vi "Select stimulus.vi"(10 "Output freq (Hz)":dbl=50.0) -> (0 "cancelled":bool, 1 "stimphases":T1, 2 "output waveform":waveform(dbl), 3 "Stimulus":T2={"type"=enum."Zero", "sinfreq start"=0.0, "sinfreq end"=0.0, "sinamp start"=0.0, "sinamp end"=0.0, "noise freq lo"=0.0, "noise freq hi"=0.0, "noiseamp start"=0.0, "noiseamp end"=0.0, "stimdur"=100.0, "before dur"=20.0, "after dur"=30.0, "pulse data"={"time"=[], "phase/vel"=[], "dir/shift"=[], "amplitude"=[], "duration"=[]}} {"noise freq hi" min=0.0 step=0.5; "noise freq lo" min=0.0 step=0.5; "noiseamp end" min=0.0 step=0.5; "noiseamp start" min=0.0 step=0.5})   [LabVIEW 2013]
uses:
  Stimulus.ctl
  Stimulus type.ctl
  Pulse data.ctl
  Stim phases.ctl
panel:
  in  "offset":dbl[unit] caption="Offset"
  out "Waveform Graph":waveform(dbl)[](graph)=[{"t0"=timestamp(0 s since 1904-01-01), "dt"=inf, "Y"=[]}, {"t0"=timestamp(0 s since 1904-01-01), "dt"=inf, "Y"=[]}, {"t0"=timestamp(0 s since 1904-01-01), "dt"=inf, "Y"=[]}]
  in  "Cancel":bool
  in  "OK":bool
  in  "Stimulus type":T5(tab)=enum."Frequency sweep"
  in  "stimdurzero":dbl=100.0 caption="Stimulus"
  in  "stimdursin":dbl=100.0 caption="Stimulus"
  in  "beforesin":dbl[unit]=20.0 caption="Before"
  in  "aftersin":dbl[unit]=30.0 caption="After"
  in  "noisehifreq":dbl[unit]=10.0 caption="High cutoff" format="%#_10g"
  in  "noiseamp":dbl[unit] caption="Amplitude"
  in  "noiselofreq":dbl[unit] caption="Low cutoff"
  in  "sinamp":dbl[unit]=0.3490658503988659 caption="Amplitude"
  in  "sinfreq":dbl[unit]=1.0 caption="Frequency" format="%#_10g"
  in  "stimdurampsweep":dbl=100.0 caption="Stimulus"
  in  "Hi freq cutoff":dbl[unit]=10.0 min=0.0 step=0.5
  in  "Lo freq cutoff":dbl[unit] min=0.0 step=0.5
  in  "Start noise":dbl[unit] caption="Start" min=0.0 step=0.008726646259971648
  in  "Frequency":dbl[unit]=1.0 min=0.0 step=0.05
  in  "Start amp":dbl[unit]=0.5235987755982988 caption="Start" min=0.0 step=0.017453292519943295
  in  "End amplitude":dbl[unit]=0.5235987755982988 caption="End" min=0.0 step=0.017453292519943295
  in  "End noise":dbl[unit] caption="End" min=0.0 step=0.008726646259971648
  in  "beforeampsweep":dbl[unit]=20.0 caption="Before"
  in  "afterampsweep":dbl[unit]=30.0 caption="After"
  in  "stimdurfreqsweep":dbl=100.0 caption="Stimulus"
  in  "beforefreqsweep":dbl[unit]=20.0 caption="Before"
  in  "afterfreqsweep":dbl[unit]=30.0 caption="After"
  in  "hi cutoff":dbl[unit]=10.0 caption="High cutoff"
  in  "noiseamp":dbl[unit] caption="Amplitude"
  in  "lo cutoff":dbl[unit] caption="Low cutoff"
  in  "endfreq":dbl[unit]=2.0 caption="End" min=0.0 step=0.05
  in  "startfreq":dbl[unit]=0.5 caption="Start" min=0.0 step=0.05
  in  "sinamp":dbl=30.0 caption="Amplitude" min=0.0 step=1.0
  in  "beforepulses":dbl[unit]=20.0 caption="Before"
  in  "afterpulses":dbl[unit]=30.0 caption="After"
  in  "precycles":dbl=1.0 caption="Initial cycles"
  out "totaltime":dbl caption="Total time"
  in  "cyclesperpulse":dbl=1.0 caption="Cycles per pulse"
  in  "pulsedur":dbl[unit]=0.02 caption="Duration"
  in  "pulseamp":dbl[unit]=0.3490658503988659 caption="Amplitude"
  in  "pulsedir":enum16{"Left", "Right", "Both"}(ring) caption="Direction"
  in  "randomphase":bool
  in  "phases":i32=1 caption="Number of phases"
  in  "pulsereps":i32=1 caption="Repetitions"
  in  "sinamp":dbl[unit]=0.3490658503988659 caption="Amplitude"
  in  "sinfreq":dbl[unit]=1.0 caption="Frequency"
  in  "rampdir":enum16{"Left", "Right", "Both"}(ring)=enum."Both" caption="Direction"
  in  "Hold time (s)":dbl[](array[numeric])=[0.0, 10.0]
  out "Total time":dbl[unit]
  in  "Randomize":bool=TRUE
  in  "Repetitions":i32=1 min=0 step=1
  in  "Final positions (deg)":dbl[](array[numeric])=[2.0, 5.0, 10.0]
  in  "Ramp velocities (deg/s)":dbl[](array[numeric])=[1.0, 10.0]
  in  "gap time (s)":dbl=5.0 min=0.0 step=0.5
  in  "beforeramps":dbl[unit]=20.0 caption="Before"
  in  "afterramps":dbl[unit]=30.0 caption="After"
  in  "beforeshifts":dbl[unit]=20.0 caption="Before"
  in  "aftershifts":dbl[unit]=30.0 caption="After"
  in  "endphases":i32=1 caption="Number of ending phases"
  in  "precycles":dbl=1.0 caption="Initial cycles"
  out "totaltime":dbl caption="Total time"
  in  "cyclespershift":dbl=1.0 caption="Cycles per stim"
  in  "shiftdur":dbl[unit]=0.02 caption="Duration"
  in  "randomize":bool
  in  "startphases":i32=1 caption="Number of starting phases"
  in  "shiftreps":i32=1 caption="Repetitions"
  in  "sinamp":dbl[unit]=0.3490658503988659 caption="Amplitude"
  in  "sinfreq":dbl[unit]=1.0 caption="Frequency"
  # "Just record baseline bursting with no stimulus"
  # "Duration:"
  # "s"
  # "Signal:"
  # "Noise:"
  # "Duration:"
  # "cycles"
  # "Signal:"
  # "Amplitude:"
  # "Noise:"
  # "Amplitude:"
  # "Duration:"
  # "cycles"
  # "Signal:"
  # "Frequency:"
  # "Noise:"
  # "Duration:"
  # "s"
  # "Signal:"
  # "Pulses:"
  # "Duration:"
  # "Signal:"
  # "Shifts:"
  # "Duration:"
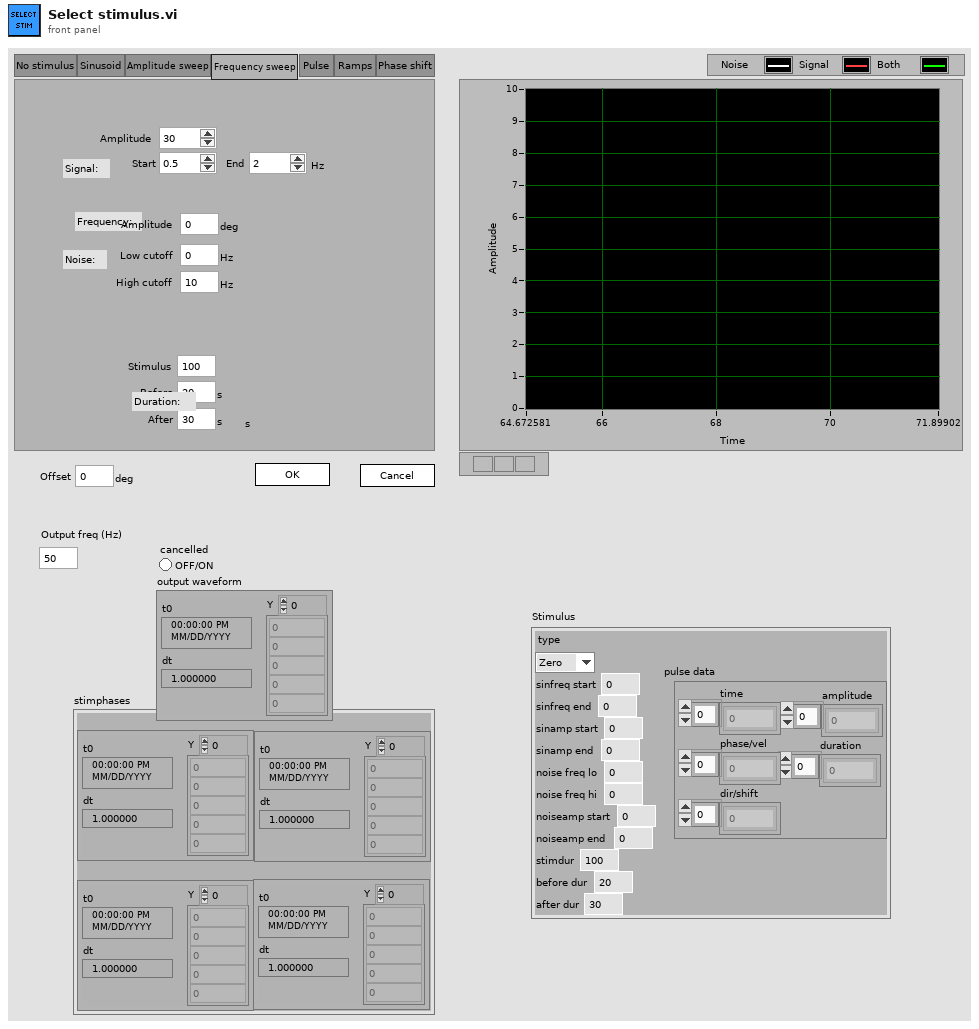
[diagram p1: front panel]
types:
  T1 = typedef "Stim phases.ctl" = cluster{"sinephase":waveform(dbl), "sinecycles":waveform(dbl), "stimphase":waveform(dbl), "stimcycles":waveform(dbl)}
  T2 = typedef "Stimulus.ctl" = cluster{"type":T3, "sinfreq start":dbl, "sinfreq end":dbl, "sinamp start":dbl, "sinamp end":dbl, "noise freq lo":dbl, "noise freq hi":dbl, "noiseamp start":dbl, "noiseamp end":dbl, "stimdur":dbl, "before dur":dbl, "after dur":dbl, "pulse data":T4}
  T3 = typedef "Stimulus type.ctl" = enum16{"Sine", "Zero", "Frequency sweep", "Two frequency", "Amplitude sweep", "Pulses", "Shifts", "Ramps"}
  T4 = typedef "Pulse data.ctl" = cluster{"time":dbl[], "phase/vel":dbl[], "dir/shift":dbl[], "amplitude":dbl[], "duration":dbl[]}
  T5 = enum32{"No stimulus", "Sinusoid", "Amplitude sweep", "Frequency sweep", "Pulse", "Ramps", "Phase shift"}
  T6 = typedef "Phases.ctl" = cluster{"sinephase":dbl[], "sinecycle":dbl[], "stimphase":dbl[], "stimcycle":dbl[]}
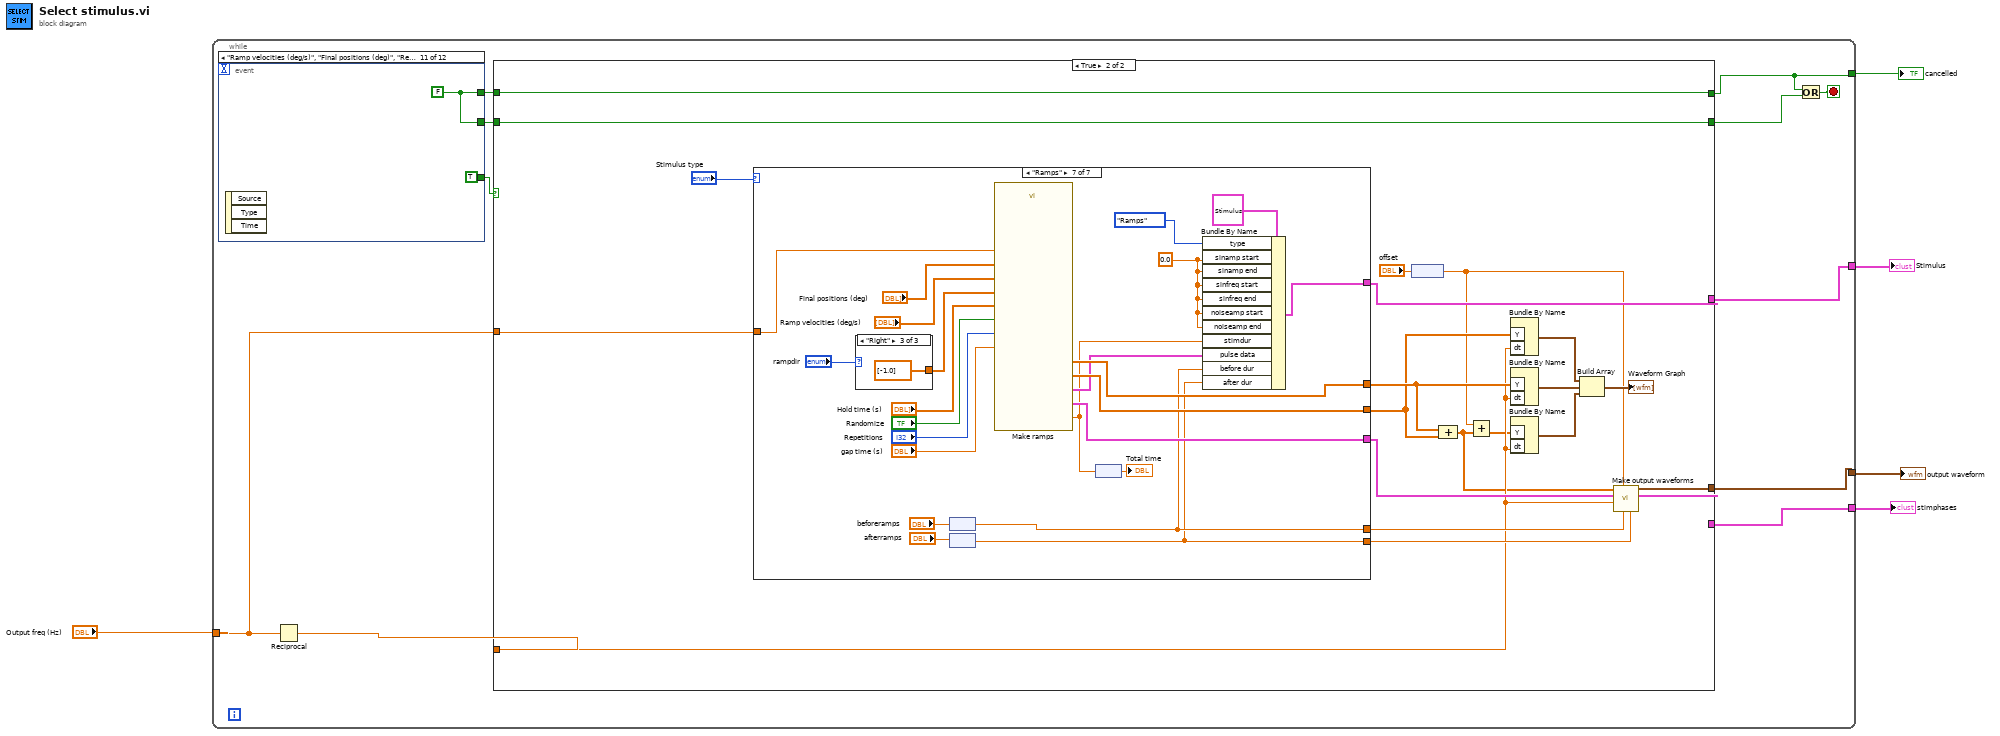
[diagram p0: block diagram]
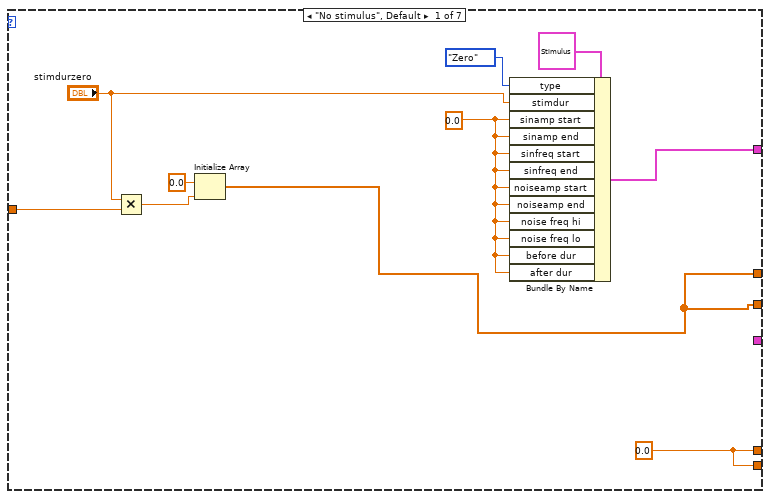
[diagram p3: hidden frame]
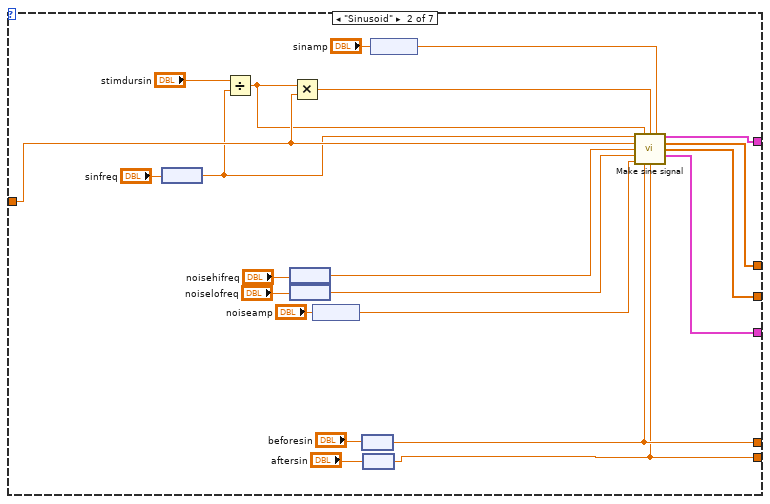
[diagram p4: hidden frame]
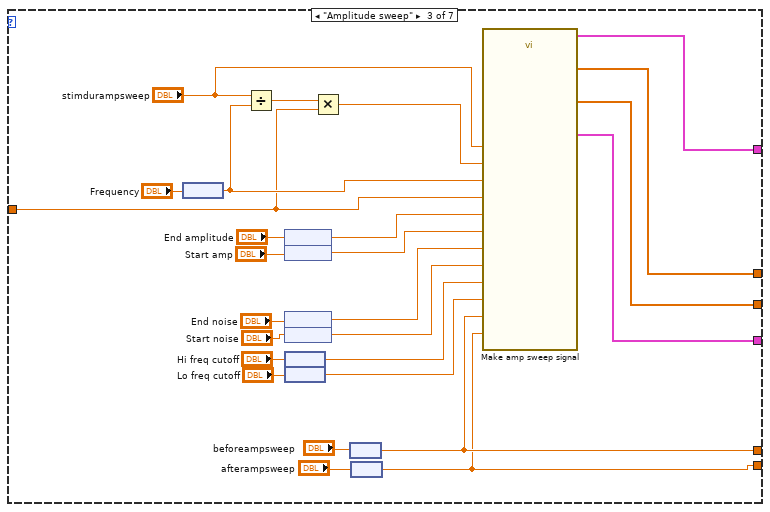
[diagram p5: hidden frame]
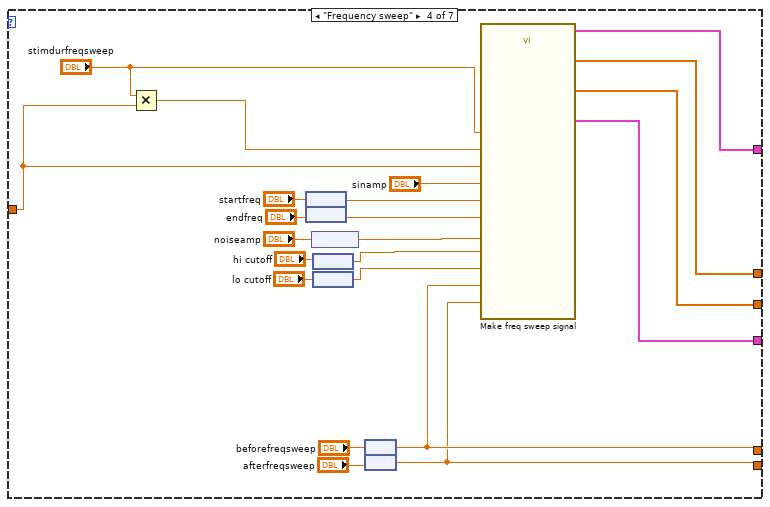
[diagram p6: hidden frame]
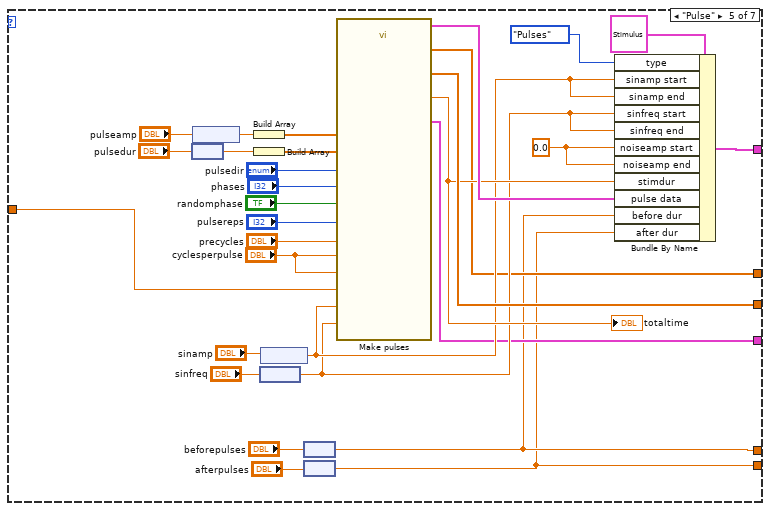
[diagram p7: hidden frame]
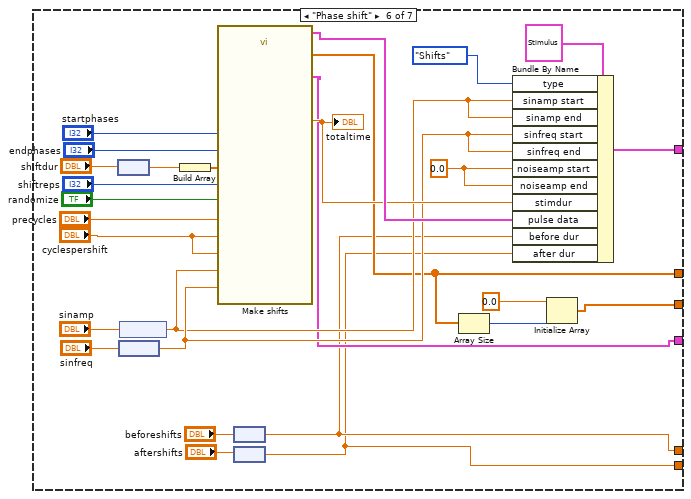
[diagram p8: hidden frame]
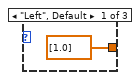
[diagram p9: hidden frame]
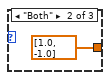
[diagram p10: hidden frame]
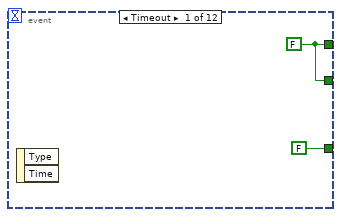
[diagram p11: hidden frame]
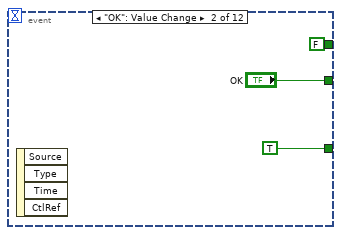
[diagram p12: hidden frame]
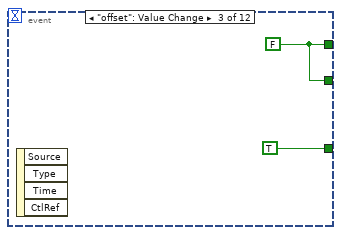
[diagram p13: hidden frame]
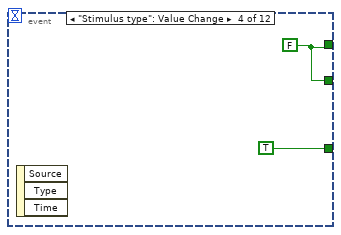
[diagram p14: hidden frame]
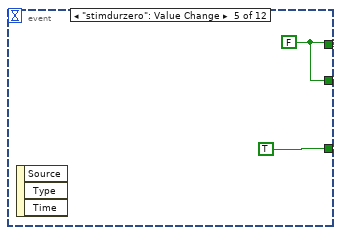
[diagram p15: hidden frame]
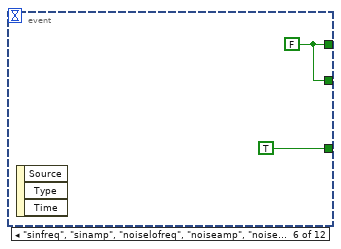
[diagram p16: hidden frame]
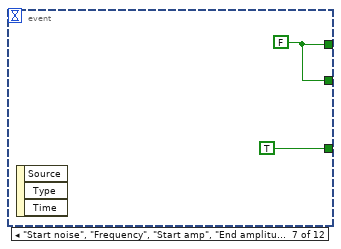
[diagram p17: hidden frame]
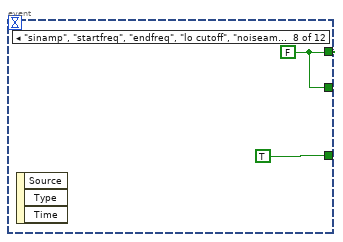
[diagram p18: hidden frame]
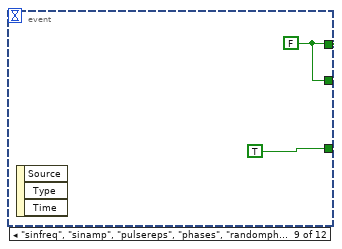
[diagram p19: hidden frame]
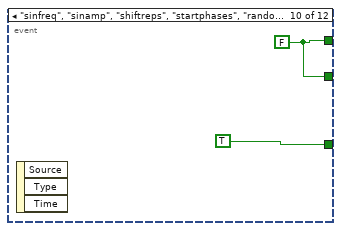
[diagram p20: hidden frame]
diagram:
  n1 = while {
    tunnel: "Output freq (Hz)" -> [w16]
    tunnel: [w7] -> w4
    tunnel: [w14] -> w3
    tunnel: [w13] -> w2
    tunnel: [w12] -> w1
    stop <- w11 stop-if-true
    n2 = event shown="[10] \"Ramp velocities (deg/s)\", \"Final positions (deg)\", \"Repetitions\", \"Randomize\", \"Hold time (s)\", \"rampdir\", \"gap time (s)\", \"beforeramps\", \"afterramps\": Value Change" {
      selector: _ -> [_ _ _ _ _ _ _ _ _ _ _ _]
      dyn-events: _ -> [_ _ _ _ _ _ _ _ _ _ _ _]
      timeout: _ -> [_ _ _ _ _ _ _ _ _ _ _ _]
      tunnel: [FALSE TRUE TRUE TRUE TRUE TRUE TRUE TRUE TRUE TRUE TRUE FALSE] -> w6
      tunnel: [w204 "OK" w209 w211 w213 w215 w217 w219 w221 w223 w226 FALSE] -> w10
      tunnel: [w204 FALSE ("Cancel") w209 w211 w213 w215 w217 w219 w221 w223 w226 "Cancel"] -> w8
      event Timeout {
        w204 = FALSE
        n3 = event-data() -> ()  [unwired: 1 in, 2 out]
      }
      event "OK": Value Change {
        n4 = event-data() -> ()  [unwired: 1 in, 4 out]
      }
      event "offset": Value Change {
        w209 = FALSE ("Cancel")
        n5 = event-data() -> ()  [unwired: 1 in, 4 out]
      }
      event "Stimulus type": Value Change {
        w211 = FALSE
        n6 = event-data() -> ()  [unwired: 1 in, 3 out]
      }
      event "stimdurzero": Value Change {
        w213 = FALSE
        n7 = event-data() -> ()  [unwired: 1 in, 3 out]
      }
      event "sinfreq", "sinamp", "noiselofreq", "noiseamp", "noisehifreq", "Hi freq cutoff", "Lo freq cutoff": Value Change {
        w215 = FALSE
        n8 = event-data() -> ()  [unwired: 1 in, 3 out]
      }
      event "Start noise", "Frequency", "Start amp", "End amplitude", "End noise": Value Change {
        w217 = FALSE
        n9 = event-data() -> ()  [unwired: 1 in, 3 out]
      }
      event "sinamp", "startfreq", "endfreq", "lo cutoff", "noiseamp", "hi cutoff": Value Change {
        w219 = FALSE
        n10 = event-data() -> ()  [unwired: 1 in, 3 out]
      }
      event "sinfreq", "sinamp", "pulsereps", "phases", "randomphase", "pulsedir", "pulseamp", "pulsedur", "cyclesperpulse", "precycles": Value Change {
        w221 = FALSE
        n11 = event-data() -> ()  [unwired: 1 in, 3 out]
      }
      event "sinfreq", "sinamp", "shiftreps", "startphases", "randomize", "shiftdur", "cyclespershift", "precycles", "endphases": Value Change {
        w223 = FALSE
        n12 = event-data() -> ()  [unwired: 1 in, 3 out]
      }
      event "Ramp velocities (deg/s)", "Final positions (deg)", "Repetitions", "Randomize", "Hold time (s)", "rampdir", "gap time (s)", "beforeramps", "afterramps": Value Change {
        w226 = FALSE ("Cancel")
        n13 = event-data() -> ()  [unwired: 1 in, 3 out]
      }
      event "Cancel": Value Change {
        n14 = event-data() -> ()  [unwired: 1 in, 5 out]
      }
    }
    n15 = Reciprocal(x=w16) -> (1/x=w15:dbl)
    n16 = case shown="True" w6 {
      tunnel: w16 -> [_ w32]
      tunnel: w15 -> [_ w28]
      tunnel: [_ w27] -> w14
      tunnel: [_ w26] -> w13
      tunnel: [_ w25] -> w12
      tunnel: w10 -> [w17 w24]
      tunnel: [w17 w24] -> w9
      tunnel: [w18 w23] -> w7
      tunnel: w8 -> [w18 w23]
      frame False {
      }
      frame True {
        n17 = case shown="\"Ramps\"" "Stimulus type" {
          tunnel: w32 -> [w48 w67 w74 w114 w132 _ w191]
          tunnel: [w40 w69 w77 w100 w126 w158 w190] -> w36
          tunnel: [w40 w64 w76 w99 w131 w156 w189] -> w35
          tunnel: [w45 w59 w78 w101 w141 w160 w180] -> w27
          tunnel: [_ w54 w75 w98 w125 w155 w187] -> w39
          tunnel: [w41 w51 w73 w103 w121 w151 w184] -> w30
          tunnel: [w41 w50 w72 w102 w120 w150 w183] -> w29
          frame "No stimulus", Default {
            w41 = 0.0
            w42 = 0.0 ("sinamp start")
            n18 = Multiply(x="stimdurzero", y=w48) -> (x*y=w47:dbl)
            n19 = Initialize Array(0.0 ("element"), w47) -> (w40:dbl[])
            n20 = Bundle By Name(cluster=T2 {"type"=enum."Zero", "sinfreq start"=0.0, "sinfreq end"=0.0, "sinamp start"=0.0, "sinamp end"=0.0, "noise freq lo"=0.0, "noise freq hi"=0.0, "noiseamp start"=0.0, "noiseamp end"=0.0, "stimdur"=0.0, "before dur"=0.0, "after dur"=0.0, "pulse data"={"time"=[], "phase/vel"=[], "dir/shift"=[], "amplitude"=[], "duration"=[]}} ("Stimulus 2"), "type"=Stimulus_type."Zero", "stimdur"="stimdurzero", "sinamp start"=w42, "sinamp end"=w42, "sinfreq start"=w42, "sinfreq end"=w42, "noiseamp start"=w42, "noiseamp end"=w42, "noise freq hi"=w42, "noise freq lo"=w42, "before dur"=w42, "after dur"=w42) -> (w45:T2)
          }
          frame "Sinusoid" {
            n21 = node("sinfreq") -> (w63:dbl)
            n22 = Divide(x="stimdursin", y=w63) -> (x/y=w58:dbl)
            n23 = node("noisehifreq") -> (w53:dbl)
            n24 = node("noiselofreq") -> (w52:dbl)
            n25 = Multiply(x=w58, y=w67) -> (x*y=w60:dbl)
            n26 = node("noiseamp") -> (w61:dbl)
            n27 = node("beforesin") -> (w51:dbl)
            n28 = node("aftersin") -> (w50:dbl)
            n29 = node("sinamp") -> (w62:dbl)
            n30 = call "Make sine signal.vi"("sinfreq"=w63, "stimdur"=w58, "nsamp"=w60, "sinamp"=w62, "Output freq (Hz)"=w67, "hicutoff"=w53, "lowcutoff"=w52, "noiseamp"=w61, "beforedur"=w51, "afterdur"=w50) -> ("Stimulus out"=w59:T2, "sine wave"=w69:dbl[], "noise"=w64:dbl[], "phases"=w54:T6)  [unwired: 2 in]
          }
          frame "Amplitude sweep" {
            n31 = node("Frequency") -> (w85:dbl)
            n32 = Divide(x="stimdurampsweep", y=w85) -> (x/y=w90:dbl)
            n33 = node("End amplitude") -> (w84:dbl)
            n34 = node("Start amp") -> (w83:dbl)
            n35 = node("End noise") -> (w82:dbl)
            n36 = node("Start noise") -> (w81:dbl)
            n37 = node("Hi freq cutoff") -> (w80:dbl)
            n38 = node("Lo freq cutoff") -> (w79:dbl)
            n39 = Multiply(x=w90, y=w74) -> (x*y=w87:dbl)
            n40 = node("beforeampsweep") -> (w73:dbl)
            n41 = node("afterampsweep") -> (w72:dbl)
            n42 = call "Make amp sweep signal.vi"("nsamp"=w87, "stimdur"="stimdurampsweep", "Output freq (Hz)"=w74, "sinfreq"=w85, "sinamp start"=w83, "sinamp end"=w84, "noiseamp start"=w81, "beforedur"=w73, "noiseamp end"=w82, "afterdur"=w72, "hicutoff"=w80, "lowcutoff"=w79) -> ("Stimulus out"=w78:T2, "sine wave"=w77:dbl[], "noise"=w76:dbl[], "phases"=w75:T6)  [unwired: 4 in]
          }
          frame "Frequency sweep" {
            n43 = Multiply(x="stimdurfreqsweep", y=w114) -> (x*y=w110:dbl)
            n44 = node("startfreq") -> (w113:dbl)
            n45 = node("endfreq") -> (w112:dbl)
            n46 = node("noiseamp") -> (w111:dbl)
            n47 = node("hi cutoff") -> (w107:dbl)
            n48 = node("lo cutoff") -> (w106:dbl)
            n49 = node("beforefreqsweep") -> (w103:dbl)
            n50 = node("afterfreqsweep") -> (w102:dbl)
            n51 = call "Make freq sweep signal.vi"("stimdurfreqsweep"="stimdurfreqsweep", "nsamp"=w110, "Output freq (Hz)"=w114, "startfreq"=w113, "endfreq"=w112, "sinamp"="sinamp", "noiseamp"=w111, "beforefreqsweep"=w103, "hicutoff"=w107, "afterfreqsweep"=w102, "lowcutoff"=w106) -> ("Stimulus"=w101:T2, "signal"=w100:dbl[], "noise"=w99:dbl[], "phases"=w98:T6)  [unwired: 5 in]
          }
          frame "Pulse" {
            w142 = 0.0 ("noiseamp start")
            n52 = node("pulsedur") -> (w146:dbl)
            n53 = node("pulseamp") -> (w148:dbl)
            n54 = Build Array(w148) -> (w140:dbl[])
            n55 = Build Array(w146) -> (w139:dbl[])
            n56 = node("sinfreq") -> (w127:dbl)
            n57 = node("sinamp") -> (w128:dbl)
            n58 = node("beforepulses") -> (w121:dbl)
            n59 = node("afterpulses") -> (w120:dbl)
            n60 = call "Make pulses.vi"("phases"="phases", "pulsedir"="pulsedir", "pulsereps"="pulsereps", "Amplitudes"=w140, "Durations"=w139, "Output freq (Hz)"=w132, "randomize"="randomphase", "pre cycles"="precycles", "post cycles"="cyclesperpulse", "cyclesperpulse"="cyclesperpulse", "sinfreq"=w127, "sinamp"=w128) -> ("pulse data"=w130:T4, "sine signal"=w126:dbl[], "pulse signal"=w131:dbl[], "totaltime"=w129:dbl, "stimphases"=w125:T6)  [unwired: 3 in]
            "totaltime" <- w129
            n61 = Bundle By Name(cluster=T2 {"type"=enum."Zero", "sinfreq start"=0.0, "sinfreq end"=0.0, "sinamp start"=0.0, "sinamp end"=0.0, "noise freq lo"=0.0, "noise freq hi"=0.0, "noiseamp start"=0.0, "noiseamp end"=0.0, "stimdur"=0.0, "before dur"=0.0, "after dur"=0.0, "pulse data"={"time"=[], "phase/vel"=[], "dir/shift"=[], "amplitude"=[], "duration"=[]}} ("Stimulus 2"), "type"=Stimulus_type."Pulses", "sinamp start"=w128, "sinamp end"=w128, "sinfreq start"=w127, "sinfreq end"=w127, "noiseamp start"=w142, "noiseamp end"=w142, "stimdur"=w129, "pulse data"=w130, "before dur"=w121, "after dur"=w120) -> (w141:T2)
          }
          frame "Phase shift" {
            w165 = 0.0 ("noiseamp start")
            n62 = node("shiftdur") -> (w177:dbl)
            n63 = node("sinfreq") -> (w162:dbl)
            n64 = node("sinamp") -> (w161:dbl)
            n65 = Build Array(w177) -> (w173:dbl[])
            n66 = call "Make shifts.vi"("startphases"="startphases", "endphases"="endphases", "pulsereps"="shiftreps", "Durations"=w173, "randomize"="randomize", "pre cycles"="precycles", "post cycles"="cyclespershift", "cyclespershift"="cyclespershift", "sinfreq"=w162, "sinamp"=w161) -> ("pulse data"=w164:T4, "sine signal"=w158:dbl[], "phases"=w155:T6, "totaltime"=w163:dbl)  [unwired: 5 in, 1 out]
            "totaltime" <- w163
            n67 = node("beforeshifts") -> (w151:dbl)
            n68 = node("aftershifts") -> (w150:dbl)
            n69 = Array Size(array=w158) -> (size(s)=w159:i32)
            n70 = Bundle By Name(cluster=T2 {"type"=enum."Zero", "sinfreq start"=0.0, "sinfreq end"=0.0, "sinamp start"=0.0, "sinamp end"=0.0, "noise freq lo"=0.0, "noise freq hi"=0.0, "noiseamp start"=0.0, "noiseamp end"=0.0, "stimdur"=0.0, "before dur"=0.0, "after dur"=0.0, "pulse data"={"time"=[], "phase/vel"=[], "dir/shift"=[], "amplitude"=[], "duration"=[]}} ("Stimulus 2"), "type"=Stimulus_type."Shifts", "sinamp start"=w161, "sinamp end"=w161, "sinfreq start"=w162, "sinfreq end"=w162, "noiseamp start"=w165, "noiseamp end"=w165, "stimdur"=w163, "pulse data"=w164, "before dur"=w151, "after dur"=w150) -> (w160:T2)
            n71 = Initialize Array(0.0 ("element"), w159) -> (w156:dbl[])
          }
          frame "Ramps" {
            w181 = 0.0
            n72 = case shown="\"Right\"" "rampdir" {
              tunnel: [dbl[] [1.0] ("Direction") dbl[] [1.0, -1.0] ("Direction") dbl[] [-1.0] ("Direction")] -> w194
              frame "Left", Default {
              }
              frame "Both" {
              }
              frame "Right" {
              }
            }
            n73 = node("beforeramps") -> (w184:dbl)
            n74 = node("afterramps") -> (w183:dbl)
            n75 = call "Make ramps.vi"("Final positions (deg)"="Final positions (deg)", "Ramp velocities (deg/s)"="Ramp velocities (deg/s)", "Direction"=w194, "Hold time (s)"="Hold time (s)", "Repetitions"="Repetitions", "randomize"="Randomize", "gap time (s)"="gap time (s)", "sampling rate"=w191) -> ("sine signal"=w190:dbl[], "ramp data"=w188:T4, "ramp signal"=w189:dbl[], "stimphases"=w187:T6, "Total time"=w182:dbl)  [unwired: 7 in]
            n76 = node(w182) -> (→"Total time":dbl[unit])
            n77 = Bundle By Name(cluster=T2 {"type"=enum."Zero", "sinfreq start"=0.0, "sinfreq end"=0.0, "sinamp start"=0.0, "sinamp end"=0.0, "noise freq lo"=0.0, "noise freq hi"=0.0, "noiseamp start"=0.0, "noiseamp end"=0.0, "stimdur"=0.0, "before dur"=0.0, "after dur"=0.0, "pulse data"={"time"=[], "phase/vel"=[], "dir/shift"=[], "amplitude"=[], "duration"=[]}} ("Stimulus 2"), "type"=Stimulus_type."Ramps", "sinamp start"=w181, "sinamp end"=w181, "sinfreq start"=w181, "sinfreq end"=w181, "noiseamp start"=w181, "noiseamp end"=w181, "stimdur"=w182, "pulse data"=w188, "before dur"=w184, "after dur"=w183) -> (w180:T2)
          }
        }
        n78 = node("offset") -> (w19:dbl)
        n79 = Compound Arithmetic op=ADD(w36, w35) -> (w21:dbl[])
        n80 = Add(x=w19, y=w21) -> (x+y=w20:dbl[])
        n81 = Bundle By Name("Y"=w35, "dt"=w28) -> (w34:waveform(dbl))  [unwired: 1 in]
        n82 = Bundle By Name("Y"=w36, "dt"=w28) -> (w37:waveform(dbl))  [unwired: 1 in]
        n83 = Bundle By Name("Y"=w20, "dt"=w28) -> (w38:waveform(dbl))  [unwired: 1 in]
        n84 = Build Array(w34, w37, w38) -> (→"Waveform Graph":waveform(dbl)[])
        n85 = call "Make output waveforms.vi"("after"=w29, "before"=w30, "offset"=w19, "dt"=w28, "stimphases in"=w39, "output"=w21) -> ("stimphases out"=w25:T1, "output waveform"=w26:waveform(dbl))  [unwired: 4 in]
      }
    }
    n86 = Or(x=w7, y=w9) -> (x .or. y?=w11:bool)
  }
  "cancelled" <- w4
  "Stimulus" <- w3
  "stimphases" <- w1
  "output waveform" <- w2
